vi "Generate Best Fit.vi"(2 "Y":dbl[](array[numeric]), 3 "X":dbl[](array[numeric])) -> (0 "Y Values":dbl[](array[numeric]), 1 "X Values":dbl[](array[numeric]))   [LabVIEW 2017]
uses:
  <vilib>/Analysis/NI_AALPro.lvlib
  <vilib>/gmath/NI_Gmath.lvlib
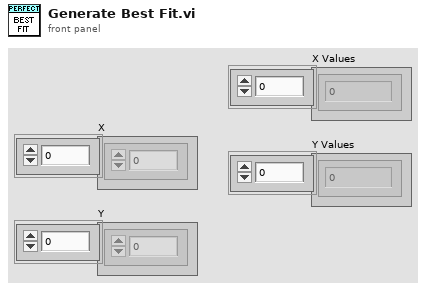
[diagram p1: front panel]
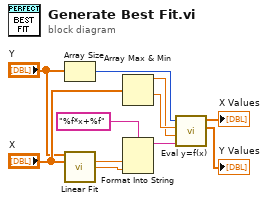
[diagram p0: block diagram]
diagram:
  n1 = Array Size(array="Y") -> (size(s)=w2:i32)
  n2 = call <vilib>:"Linear Fit.vi"("Y"="Y", "X"="X") -> ("slope"=w10:dbl, "intercept"=w4:dbl)  [unwired: 9 in, 3 out]
  n3 = Array Max & Min(array="X") -> (max value=w8:dbl, min value=w9:dbl)  [unwired: 2 out]
  n4 = Format Into String(format string="%f*x+%f", w10, w4) -> (resulting string=w5:string)  [unwired: 2 in, 1 out]
  n5 = call <vilib>:"Eval y=f(x).vi"("formula"=w5, "end"=w8, "start"=w9, "number of points"=w2) -> ("Y Values"=→"Y Values":dbl[], "X Values"=→"X Values":dbl[])  [unwired: 2 out]
